vi "Read all.vi"(0 "Овны":refnum<class "Modbus Master.lvclass">[](array[class]), 1 "3-регистра(501)":u16[](array[numeric]), 5 "Клапана":bool[](array[boolean]), 11 "error in (no error)":errorcluster) -> (4 "Овны 2":refnum<class "Modbus Master.lvclass">[](array[class]), 6 "Р пластовое":sgl format="%#.4f", 8 "Р горное":sgl format="%#.4f", 10 "Din":bool[](array[boolean]), 13 "Р атм.":sgl format="%#.4f", 14 "Температура":sgl format="%#.4f", 15 "error out":errorcluster)   [LabVIEW 2018]
uses:
  <vilib>/NI/Modbus Library/API/Master/Modbus Master.lvclass
  C:/Program Files (x86)/National Instruments/LabVIEW 2018/vi.lib/NI/Modbus Library/API/Modbus API.lvclass
panel:
  out "4входа(4-20)101":u16[](array[numeric])
  out "register 51":u16[](array[numeric])
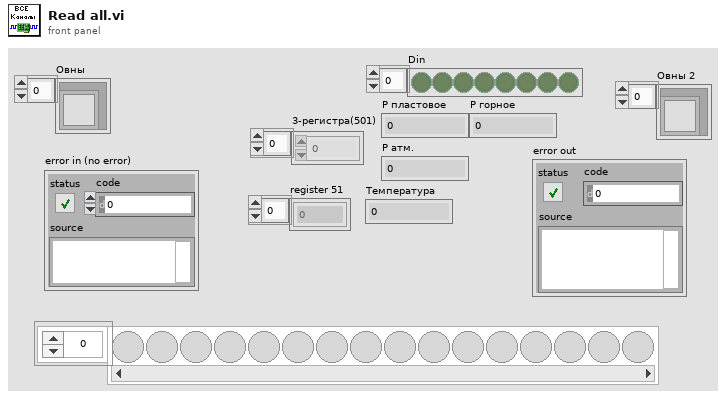
[diagram p1: front panel]
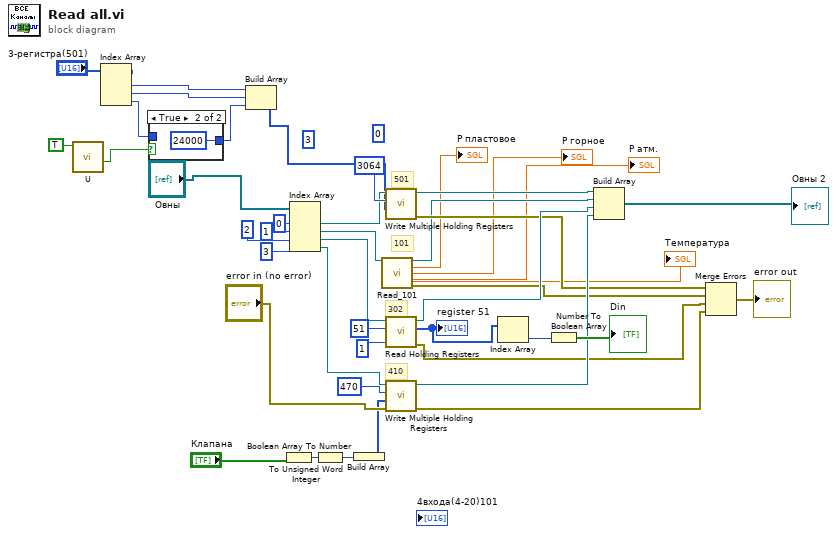
[diagram p0: block diagram]
diagram:
  (unwired) u16 3 ("quantity")
  (unwired) u16 0 ("holding register value")
  # "410"
  # "302"
  # "101"
  # "501"
  n1 = call "U.vi"("Boolean"=TRUE) -> ("x = y?"=w1:bool)  [unwired: 10 in]
  n2 = Index Array(array="3-регистра(501)") -> (element #1=w6:u16, element #2=w7:u16, element #3=w4:u16)  [unwired: 3 in]
  n3 = case shown="True" w1 {
    tunnel: w4 -> [w44 _]
    tunnel: [w44 u16 24000 ("Register")] -> w3
    frame False {
    }
    frame True {
    }
  }
  n4 = Build Array(w6, w7, w3) -> (w2:u16[])
  n5 = Boolean Array To Number(Boolean array="Клапана") -> (number=w26:u32)
  n6 = Index Array(array="Овны", index #1=0 ("index"), index #2=1 ("index"), index #3=2 ("index"), index #4=3 ("index")) -> (element #1=w24:refnum<class "Modbus Master.lvclass">, element #2=w16:refnum<class "Modbus Master.lvclass">, element #3=w36:refnum<class "Modbus Master.lvclass">, element #4=w40:refnum<class "Modbus Master.lvclass">)
  n7 = To Unsigned Word Integer(number=w26) -> (unsigned 16bit integer=w20:u16)
  n8 = Build Array(w20) -> (w19:u16[])
  n9 = call "Read_101.vi"("Modbus instance in"=w16) -> ("Modbus instance out"=w15:refnum<class "Modbus Master.lvclass">, "Р пластовое"=→"Р пластовое":sgl, "Р горное"=→"Р горное":sgl, "Р атм."=→"Р атм.":sgl, "Температура"=→"Температура":sgl, "error out"=w14:errorcluster)  [unwired: 9 in]
  n10 = call-dynamic "Write Multiple Holding Registers.vi"("registers to write"=w2, "starting address"=u16 3064 ("address"), "Modbus master in"=w24) -> ("error out"=w22:errorcluster, "Modbus master out"=w23:refnum<class "Modbus Master.lvclass">)  [unwired: 7 in]
  n11 = call-dynamic "Read Holding Registers.vi"("number of inputs"=u16 1 ("number of holding registers"), "starting address"=u16 51, "Modbus master in"=w36) -> ("error out"=w30:errorcluster, "register values"=w41:u16[], "Modbus master out"=w32:refnum<class "Modbus Master.lvclass">)  [unwired: 6 in]
  "register 51" <- w41
  n12 = call-dynamic "Write Multiple Holding Registers.vi"("error in"="error in (no error)", "registers to write"=w19, "starting address"=u16 470 ("address"), "Modbus master in"=w40) -> ("error out"=w29:errorcluster, "Modbus master out"=w31:refnum<class "Modbus Master.lvclass">)  [unwired: 6 in]
  n13 = Index Array(array=w41) -> (element=w42:u16)  [unwired: 1 in]
  n14 = Number To Boolean Array(number=w42) -> (Boolean array=→"Din":bool[])
  n15 = Build Array(w23, w15, w32, w31) -> (→"Овны 2":refnum<class "Modbus Master.lvclass">[])
  n16 = Merge Errors(w22, w14, w30, w29) -> (→"error out":errorcluster)
